vi "CallGraphAttr.vi"(10 "Event In":refnum<class "NISAST Event.lvclass">, 11 "名称或相对路径":string="GraphAttribute.vi") -> ()   [LabVIEW 2012, in "WaveGraphX.xctl"]
uses:
  WaveGraphX.xctl
  <resource>/importtools/Common/Event/NISAST Event.lvclass
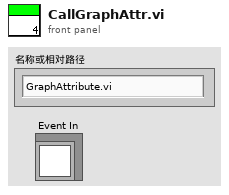
[diagram p1: front panel]
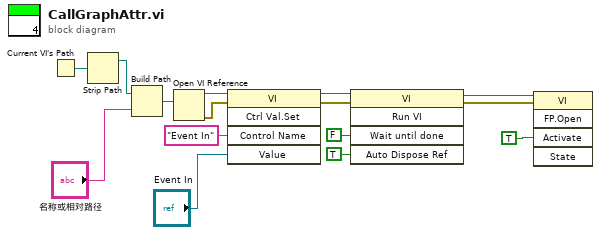
[diagram p0: block diagram]
diagram:
  n1 = Current VI's Path() -> (path=w8:path)
  n2 = Strip Path(path=w8) -> (stripped path=w7:path)  [unwired: 1 out]
  n3 = Build Path(base path=w7, name or relative path="名称或相对路径") -> (appended path=w10:path)
  n4 = Open VI Reference(vi path=w10) -> (vi reference=w11:refnum<vi>, error out=w12:errorcluster)  [unwired: 5 in]
  n5 = invoke class="VI" method="Ctrl Val.Set"(reference=w11, error in=w12, "Control Name"="Event In" ("控件名"), "Value"="Event In") -> (reference out=w13:refnum<vi>, error out=w14:errorcluster)  [unwired: 1 in, 3 out]
  n6 = invoke class="VI" method="Run VI"(reference=w13, error in=w14, "Wait until done"=FALSE ("结束前等待"), "Auto Dispose Ref"=TRUE ("自动销毁引用")) -> (reference out=w6:refnum<vi>, error out=w5:errorcluster)  [unwired: 1 in, 3 out]
  n7 = invoke class="VI" method="FP.Open"(reference=w6, error in=w5, "Activate"=TRUE ("激活？")) -> ()  [unwired: 2 in, 5 out]
